vi "StrChange.vi"(8 "error in":errorcluster caption="错误输入", 11 "StrIn":string="80:C5:F2:7F:6F:CD") -> (0 "error out":errorcluster caption="错误输出", 3 "StrOut":string)   [LabVIEW 2013]
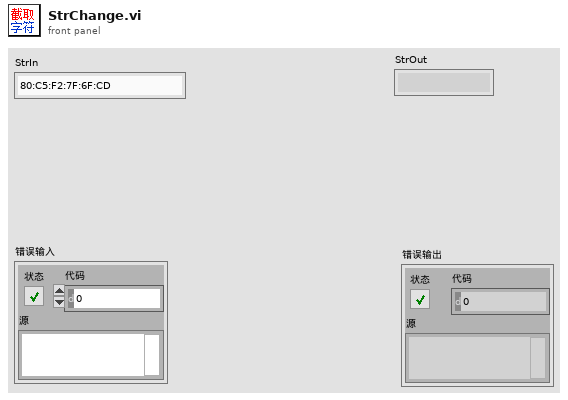
[diagram p1: front panel]
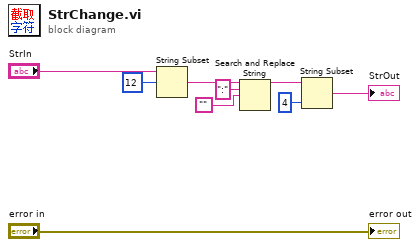
[diagram p0: block diagram]
diagram:
  n1 = String Subset(string="StrIn", offset (0)=12 ("长度（剩余）")) -> (substring=w7:string)  [unwired: 1 in]
  n2 = Search and Replace String(input string=w7, search string=":" ("搜索字符串"), replace string="") -> (result string=w4:string)  [unwired: 5 in, 3 out]
  n3 = String Subset(string=w4, length (rest)=4 ("长度（剩余）")) -> (substring=→"StrOut":string)  [unwired: 1 in]
  "error out" <- "error in"
